vi "Do.vi"(8 "error in (no error)":errorcluster, 10 "Actor in":refnum<class "Actor.lvclass">, 11 "Log Status":refnum<class "Log Status.lvclass">) -> (0 "error out":errorcluster, 2 "Actor out":refnum<class "Actor.lvclass">)   [LabVIEW 2015, in "Controller Actor.lvlib" / "Log Status.lvclass"]
uses:
  Log Status.lvclass
  <vilib>/ActorFramework/Actor/Actor.lvclass
  Controller.lvclass
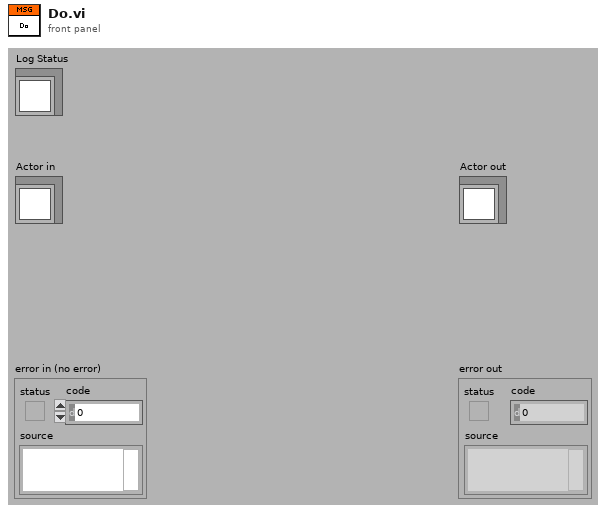
[diagram p1: front panel]
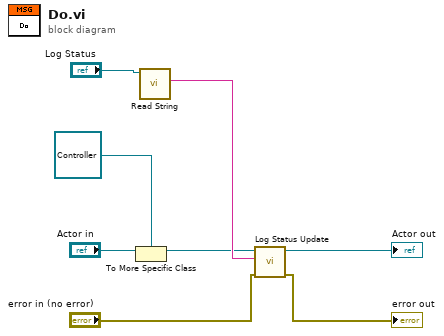
[diagram p0: block diagram]
diagram:
  n1 = To More Specific Class(target class=refnum<class "Controller.lvclass"> refnum ("Controller.lvclass"), reference="Actor in") -> (specific class reference=w4:refnum<class "Controller.lvclass">)  [unwired: 1 in, 1 out]
  n2 = call "Read String.vi"("Log Status in"="Log Status") -> ("String"=w5:string)  [unwired: 8 in, 2 out]
  n3 = call-dynamic "Log Status Update.vi"("error in (no error)"="error in (no error)", "String"=w5, "Controller in"=w4) -> ("error out"=→"error out":errorcluster, "Controller out"=→"Actor out":refnum<class "Controller.lvclass">)  [unwired: 7 in]
